vi "Teleop.vi"(10 "Match Info":T1={"Autonomous Elapsed Seconds"=0.0, "TeleOp Elapsed Seconds"=0.0, "Disabled Elapsed Seconds"=0.0, "Visited Autonomous"=FALSE, "Visited TeleOp"=FALSE, "Visited Disabled"=FALSE, "Autonomous Settings"={"Autonomous Style"=enum."Independent", "VI Refnum"=refnum}}, 11 "Call Context":T2) -> ()   [LabVIEW 2014]
doc: "This VI is called for each TeleOp packet received from the DS where the robot is not disabled. It is often used to read from the joysticks and update I/O or to update setpoints for timed control loops. It should complete and return within 20 milliseconds or it may miss DS packets."
uses:
  <vilib>/Rock Robotics/WPI/DriverStation/WPI_DriverStationDerivedRobotMode.ctl
  <vilib>/Rock Robotics/WPI/DriverStation/WPI_DriverStationMatch Info.ctl
  Global Variables.vi
  <vilib>/Rock Robotics/WPI/Joystick/WPI_JoystickGetSetRefNum.vi
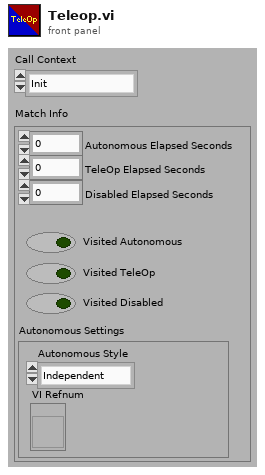
[diagram p1: front panel]
types:
  T1 = typedef "WPI_DriverStationMatch Info.ctl" = cluster{"Autonomous Elapsed Seconds":dbl, "TeleOp Elapsed Seconds":dbl, "Disabled Elapsed Seconds":dbl, "Visited Autonomous":bool, "Visited TeleOp":bool, "Visited Disabled":bool, "Autonomous Settings":cluster{"Autonomous Style":enum16{"Iterative", "Independent"}, "VI Refnum":refnum<vi>}}
  T2 = typedef "WPI_DriverStationDerivedRobotMode.ctl" = enum16{"Init", "Execute", "Stop"}
  T3 = typedef "WPI_JoystickDevRef.ctl" = cluster{"Device":T4}
  T4 = typedef "WPI_JoystickDeviceEnum.ctl" = enum16{"USB 0", "USB 1", "USB 2", "USB 3", "USB 4", "USB 5"}
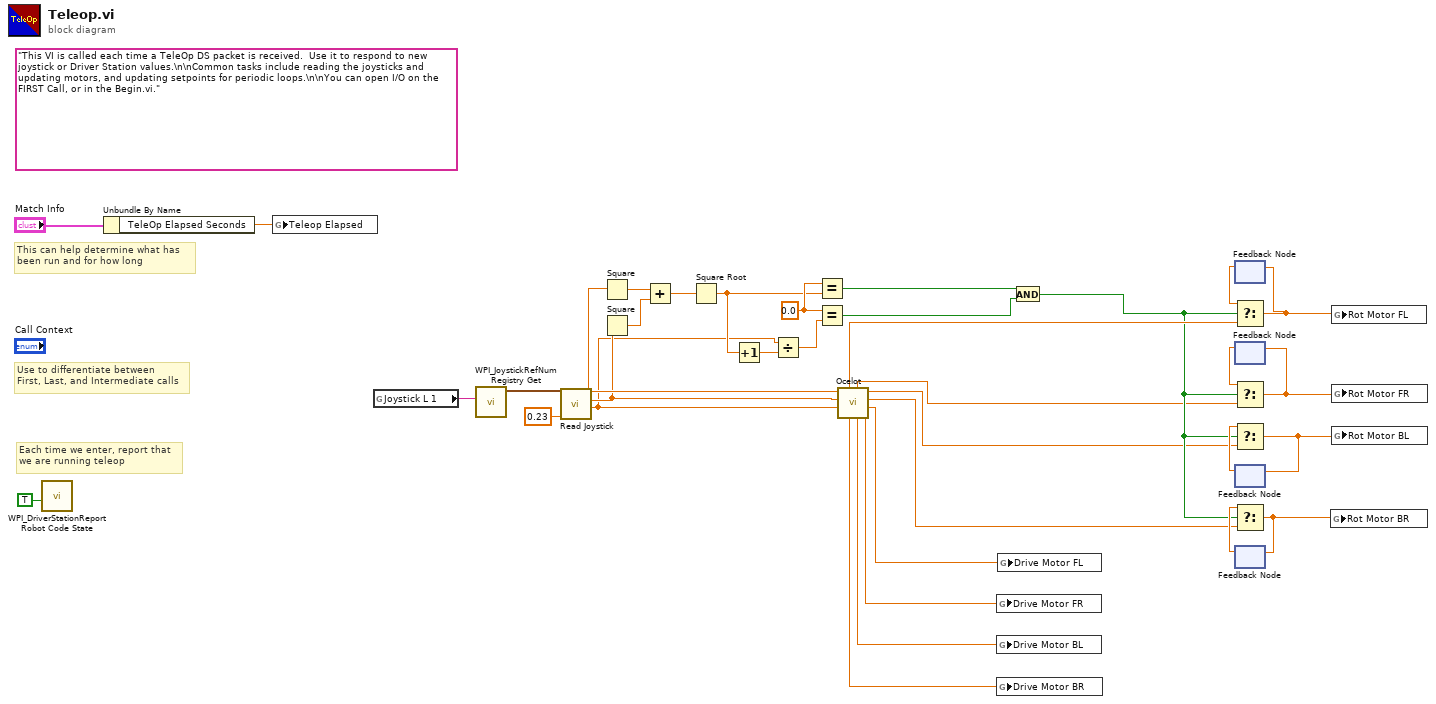
[diagram p0: block diagram]
diagram:
  w27 = 0.0 ("x")
  (unwired) "This VI is called each time a TeleOp DS packet is received.  Use it to respond to new joystick or Driver Station values.\n\nCommon tasks include reading the joysticks and updating motors, and updating setpoints for periodic loops.\n\nYou can open I/O on the FIRST Call, or in the Begin.vi."
  # "Each time we enter, report that\nwe are running teleop"
  # "Use to differentiate between\nFirst, Last, and Intermediate calls"
  # "This can help determine what has\nbeen run and for how long"
  n1 = call <vilib>:"WPI_DriverStationReport Robot Code State.vi"("TeleOp"=TRUE ("Autonomous")) -> ()  [unwired: 10 in, 1 out]
  n2 = Unbundle By Name("Match Info") -> ("TeleOp Elapsed Seconds"=w1:dbl)
  n3 = global write "Global Variables.vi" "Teleop Elapsed"(w1) -> ()
  n4 = global read "Global Variables.vi" "Joystick L 1"() -> (w33:string)
  n5 = call <vilib>:"WPI_JoystickRefNum Registry Get.vi"("refnum name"=w33) -> ("JoystickDevRef"=w32:T3)  [unwired: 1 in, 9 out]
  n6 = call "Read Joystick.vi"("Joystick Deadbanded Value (default of 0.1)"=0.23, "Joystick L 1 DevRef"=w32) -> ("Joystick L 2 X Axis"=w2:dbl, "Joystick L 1 Y Axis"=w3:dbl, "Joystick L 1 X Axis"=w4:dbl)  [unwired: 7 in]
  n7 = Square(x=w4) -> (x^2=w29:dbl)
  n8 = Square(x=w3) -> (x^2=w30:dbl)
  n9 = Add(x=w29, y=w30) -> (x+y=w28:dbl)
  n10 = Square Root(x=w28) -> (sqrt(x)=w26:dbl)
  n11 = Increment(x=w26) -> (x+1=w25:dbl)
  n12 = Divide(x=w2, y=w25) -> (x/y=w24:dbl)
  n13 = Equal?(x=w27, y=w26) -> (x = y?=w18:bool)
  n14 = Equal?(x=w27, y=w24) -> (x = y?=w17:bool)
  n15 = call "Ocelot.vi"("RCW (X2)"=w2, "FWD (Y)"=w3, "STR (X)"=w4) -> ("FRD"=w7:dbl, "FLD"=w8:dbl, "BRS"=w9:dbl, "BLS"=w10:dbl, "BLD"=w6:dbl, "FRS"=w11:dbl, "BRD"=w5:dbl, "FLS"=w19:dbl)  [unwired: 1 in]
  n16 = global write "Global Variables.vi" "Drive Motor FR"(w7) -> ()
  n17 = global write "Global Variables.vi" "Drive Motor BL"(w6) -> ()
  n18 = global write "Global Variables.vi" "Drive Motor BR"(w5) -> ()
  n19 = global write "Global Variables.vi" "Drive Motor FL"(w8) -> ()
  n20 = And(x=w18, y=w17) -> (x .and. y?=w16:bool)
  n21 = feedback #1() -> (w23:dbl)  [unwired: 1 in]
  n22 = Select(t=w23, s=w16, f=w19) -> (s? t:f=w15:dbl)
  n23 = feedback-in #1(w15) -> ()
  n24 = feedback #2() -> (w22:dbl)  [unwired: 1 in]
  n25 = Select(t=w22, s=w16, f=w11) -> (s? t:f=w14:dbl)
  n26 = feedback-in #2(w14) -> ()
  n27 = feedback #3() -> (w21:dbl)  [unwired: 1 in]
  n28 = Select(t=w21, s=w16, f=w10) -> (s? t:f=w13:dbl)
  n29 = feedback-in #3(w13) -> ()
  n30 = feedback #4() -> (w20:dbl)  [unwired: 1 in]
  n31 = Select(t=w20, s=w16, f=w9) -> (s? t:f=w12:dbl)
  n32 = feedback-in #4(w12) -> ()
  n33 = global write "Global Variables.vi" "Rot Motor BR"(w12) -> ()
  n34 = global write "Global Variables.vi" "Rot Motor FL"(w15) -> ()
  n35 = global write "Global Variables.vi" "Rot Motor FR"(w14) -> ()
  n36 = global write "Global Variables.vi" "Rot Motor BL"(w13) -> ()
